vi "LoginTest.vi"() -> ()   [LabVIEW 2020]
uses:
  Person_List/PL_Global.vi
panel:
  in  "pwl":i32
  in  "unl":i32
  in  "OK Button":bool
  in  "PASSWORD":string
  in  "USERNAME":string
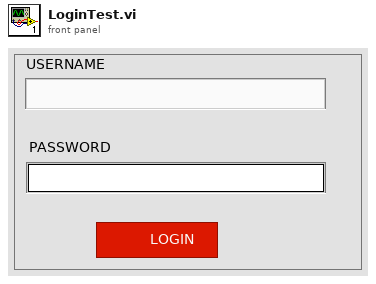
[diagram p1: front panel]
types:
  T1 = cluster{"NAMES":string[], "ID":dbl[], "PASSWORD":string[]}
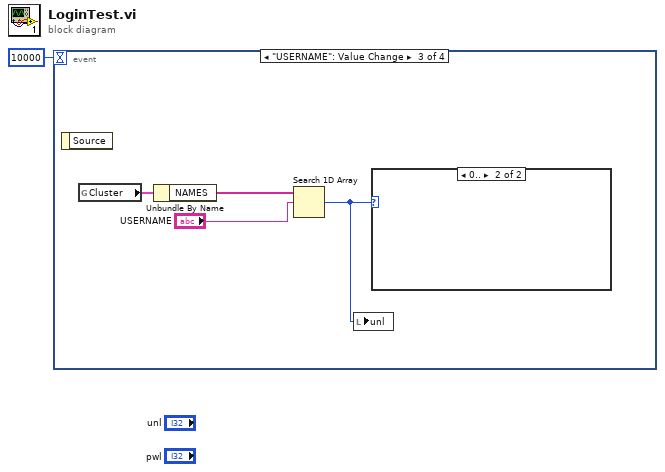
[diagram p0: block diagram]
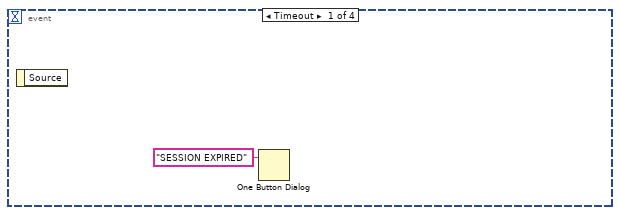
[diagram p2: hidden frame]
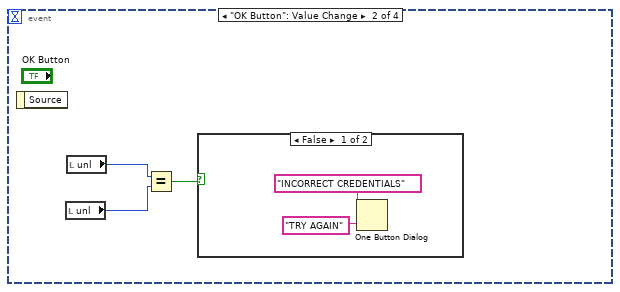
[diagram p3: hidden frame]
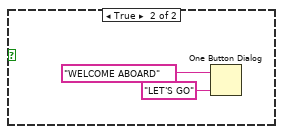
[diagram p4: hidden frame]
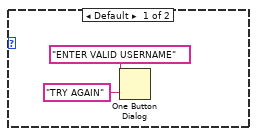
[diagram p5: hidden frame]
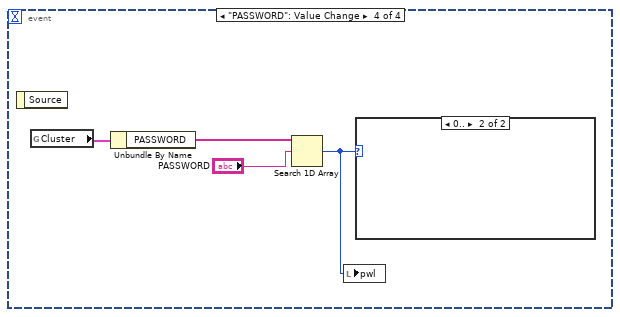
[diagram p6: hidden frame]
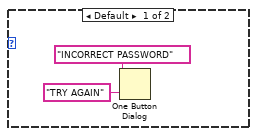
[diagram p7: hidden frame]
diagram:
  n1 = event shown="[2] \"USERNAME\": Value Change" {
    selector: _ -> [_ _ _ _]
    dyn-events: _ -> [_ _ _ _]
    timeout: 10000 -> [_ _ _ _]
    event Timeout {
      n2 = event-data() -> ()  [unwired: 1 in, 1 out]
      n3 = One Button Dialog(message="SESSION EXPIRED") -> ()  [unwired: 1 in, 1 out]
    }
    event "OK Button": Value Change {
      n4 = event-data() -> ()  [unwired: 1 in, 1 out]
      n5 = local read "unl"() -> (w3:i32)
      n6 = local read "unl"() -> (w4:i32)
      n7 = Equal?(x=w4, y=w3) -> (x = y?=w5:bool)
      n8 = case shown="False" w5 {
        frame False {
          n9 = One Button Dialog(message="INCORRECT CREDENTIALS", button name ("OK")="TRY AGAIN") -> ()  [unwired: 1 out]
        }
        frame True {
          n10 = One Button Dialog(message="WELCOME ABOARD", button name ("OK")="LET'S GO") -> ()  [unwired: 1 out]
        }
      }
    }
    event "USERNAME": Value Change {
      n11 = event-data() -> ()  [unwired: 1 in, 1 out]
      n12 = global read "PL_Global.vi" "Cluster"() -> (w13:T1)
      n13 = Unbundle By Name(w13) -> ("NAMES"=w12:string[])
      n14 = Search 1D Array(1D array=w12, element="USERNAME") -> (index of element=w10:i32)  [unwired: 1 in]
      n15 = local write "unl"(w10) -> ()
      n16 = case shown="0.." w10 {
        frame Default {
          n17 = One Button Dialog(message="ENTER VALID USERNAME", button name ("OK")="TRY AGAIN") -> ()  [unwired: 1 out]
        }
        frame 0.. {
        }
      }
    }
    event "PASSWORD": Value Change {
      n18 = event-data() -> ()  [unwired: 1 in, 1 out]
      n19 = global read "PL_Global.vi" "Cluster"() -> (w19:T1)
      n20 = Unbundle By Name(w19) -> ("PASSWORD"=w18:string[])
      n21 = Search 1D Array(1D array=w18, element="PASSWORD") -> (index of element=w16:i32)  [unwired: 1 in]
      n22 = local write "pwl"(w16) -> ()
      n23 = case shown="0.." w16 {
        frame Default {
          n24 = One Button Dialog(message="INCORRECT PASSWORD", button name ("OK")="TRY AGAIN") -> ()  [unwired: 1 out]
        }
        frame 0.. {
        }
      }
    }
  }
